vi "Ramp.vi"(1 "Speed increment":dbl, 2 "last speed":dbl, 3 "Joystick speed":dbl) -> (0 "speed setting":dbl)   [LabVIEW 2011]
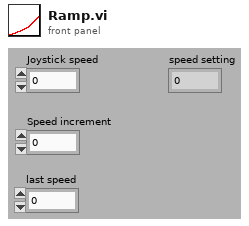
[diagram p1: front panel]
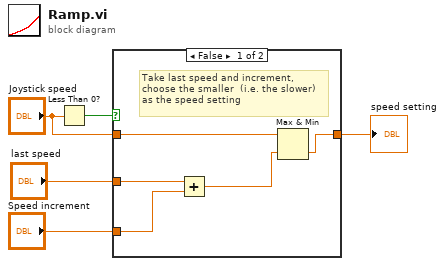
[diagram p0: block diagram]
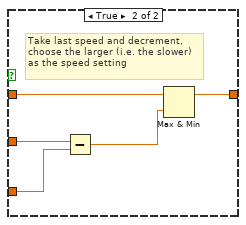
[diagram p2: hidden frame]
diagram:
  n1 = Less Than 0?(x="Joystick speed") -> (x < 0?=w3:bool)
  n2 = case shown="False" w3 {
    tunnel: "Speed increment" -> [w7 w12]
    tunnel: "Joystick speed" -> [w9 w15]
    tunnel: [w8 w13] -> w2
    tunnel: "last speed" -> [w6 w11]
    frame False {
      # "Take last speed and increment,\nchoose the smaller  (i.e. the slower)\nas the speed setting"
      n3 = Add(x=w6, y=w7) -> (x+y=w10:dbl)
      n4 = Max & Min(x=w9, y=w10) -> (min(x,y)=w8:dbl)  [unwired: 1 out]
    }
    frame True {
      # "Take last speed and decrement,\nchoose the larger (i.e. the slower)\nas the speed setting"
      n5 = Subtract(x=w11, y=w12) -> (x-y=w14:dbl)
      n6 = Max & Min(x=w15, y=w14) -> (max(x,y)=w13:dbl)  [unwired: 1 out]
    }
  }
  "speed setting" <- w2
